vi "Convert State For Save.vi"(8 "error in (no error)":errorcluster, 10 "Container State":T1, 11 "Display State":T2={"Buttons Displayed"=0, "Button States"=[], "Button Size"=0, "Button Style"=enum."Classic", "Active Button"=0, "Force Regen?"=FALSE, "Tip String Ref"=refnum}) -> (0 "error out":errorcluster, 3 "Display State To Save":variant)   [LabVIEW 2012, in "Toolbar.xctl"]
doc: "Just make sure we've pulled the volatile state into the state cluster before saving"
uses:
  Toolbar.xctl
  Toolbar State.ctl
  Button_Class/Button.lvclass
  Button_Class/Type Defs/Button Style.ctl
  <vilib>/_xctls/Container State.ctl
  <vilib>/_xctls/XControlSupport.lvlib
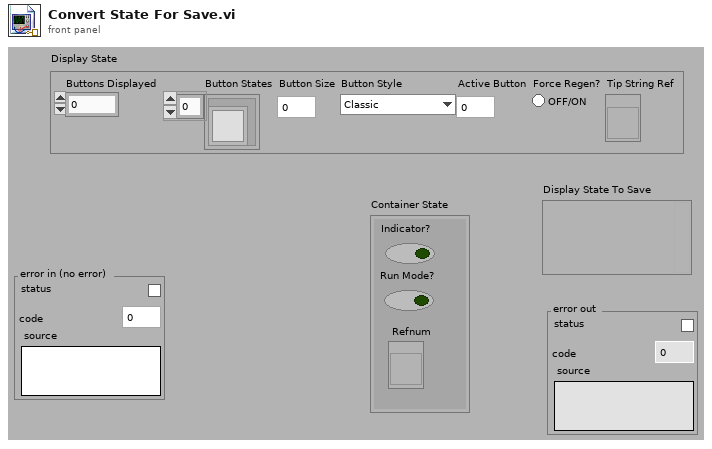
[diagram p1: front panel]
types:
  T1 = typedef "XControlSupport.lvlib/Container State.ctl" = cluster{"Indicator?":bool, "Run Mode?":bool, " Refnum":refnum<vi>}
  T2 = typedef "Toolbar.xctl/Toolbar State.ctl" = cluster{"Buttons Displayed":i32, "Button States":refnum<class "Button.lvclass">[], "Button Size":i32, "Button Style":T3, "Active Button":i32, "Force Regen?":bool, "Tip String Ref":refnum<vi>}
  T3 = typedef "Button.lvclass/Button Style.ctl" = enum16{"System", "Modern", "Classic", "Rounded", "Silver", "Ni Theme", "Metallic"}
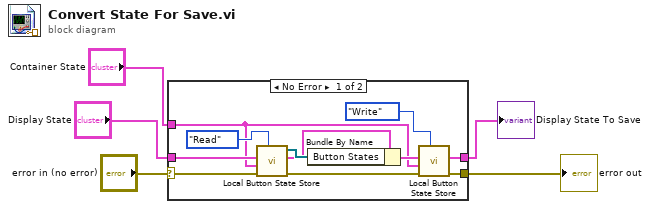
[diagram p0: block diagram]
diagram:
  n1 = case shown="No Error" "error in (no error)" {
    selector: "error in (no error)" -> [w7 w18]
    tunnel: "Display State" -> [w14 w17]
    tunnel: [w11 w17] -> w4
    tunnel: "Container State" -> [w9 _]
    tunnel: [w6 w18] -> w1
    frame No Error {
      n2 = call "Local Button State Store.vi"("Operation"=enum16{"Read", "Write"}."Read", "error in (no error)"=w7, "Container State"=w9, "Display State In"=w14) -> ("error out"=w8:errorcluster, "Display State Out"=w13:T2, "Button States"=w15:refnum<class "Button.lvclass">[])  [unwired: 5 out]
      n3 = Bundle By Name(cluster=w13, "Button States"=w15) -> (w12:T2)
      n4 = call "Local Button State Store.vi"("Operation"=enum16{"Read", "Write"}."Write", "error in (no error)"=w8, "Container State"=w9, "Display State In"=w12) -> ("error out"=w6:errorcluster, "Display State Out"=w11:T2)  [unwired: 6 out]
    }
    frame Error {
    }
  }
  "Display State To Save" <- w4
  "error out" <- w1
